vi "Master_Reader_StateMachine.vi"() -> ()   [LabVIEW 2016]
panel:
  in  "Data Directory Path":path
  in  "Directory Tree":string[](tree)
  out "arrof filesboi":path[](array[path])
  in  "Parse File / Folder":bool
  in  "target file / folder":path=path "C:/"
  in  "EXIT BUTTON":bool
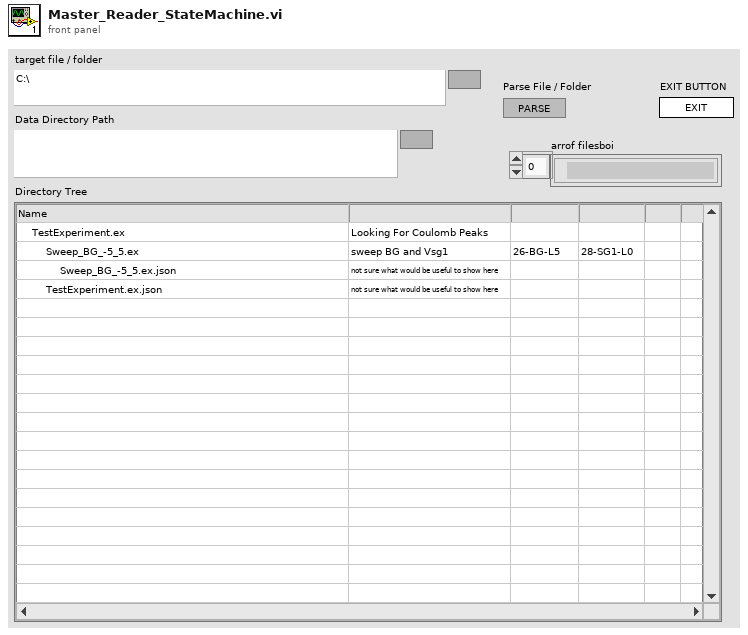
[diagram p1: front panel]
types:
  T1 = enum32{"invalid app kind", "Development System", "Run Time System", "Student Edition", "Embedded LabVIEW", "Evaluation", "Custom"}
  T2 = enum32{"Invalid", "Standard", "Closed", "Hidden", "Minimized", "Maximized"}
  T3 = cluster{"Core":cluster{"Current VI Reference":refnum<vi>, "Close Panel on Exit?":bool}, "array of files":path[], "Array of ITX Clusters ":cluster{"wave names":string[], "last modified timestamp":timestamp, "Comments":string, "Array of clusters of wave data":cluster{"wave data":dbl[]}[]}[], "target file / folder":path}
  T4 = cluster{"wave names":string[], "last modified timestamp":timestamp, "Comments":string, "Array of clusters of wave data":cluster{"wave data":dbl[]}[]}[]
  T5 = cluster{"Current VI Reference":refnum<vi>, "Close Panel on Exit?":bool}
  T6 = cluster{"wave names":string[], "last modified timestamp":timestamp, "Comments":string, "Array of clusters of wave data":cluster{"wave data":dbl[]}[]}
  T7 = typedef "imagedata.ctl" = cluster{"image type":i32, "image depth":i32, "image":u8[], "mask":u8[], "colors":u32[], "Rectangle":cluster{"left":i16, "top":i16, "right":i16, "bottom":i16}}
  T8 = cluster{"Left Cell String":string, "Child Text":string[], "Child Tag":string, "Item Indent":i32, "Child Only?":bool, "Glyph Index":i32}[]
  T9 = cluster{"Left Cell String":string, "Child Text":string[], "Child Tag":string, "Item Indent":i32, "Child Only?":bool, "Glyph Index":i32}
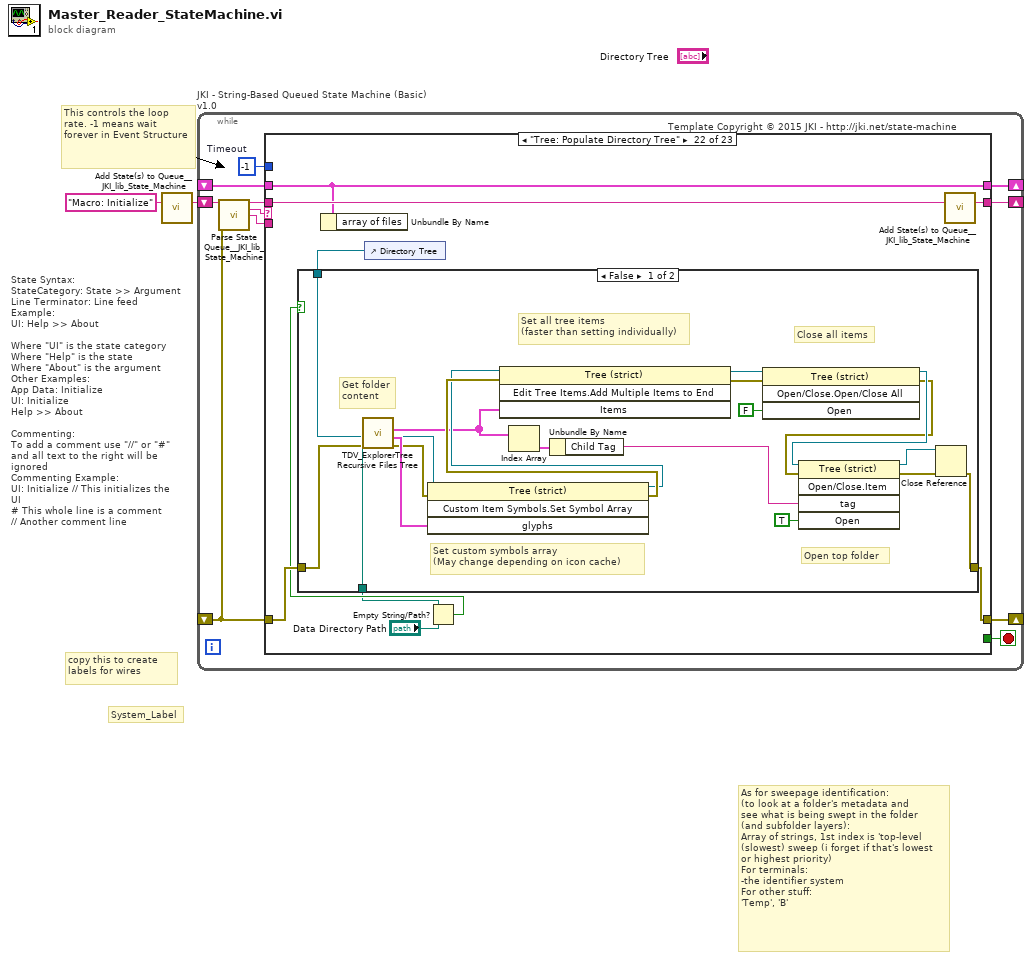
[diagram p0: block diagram]
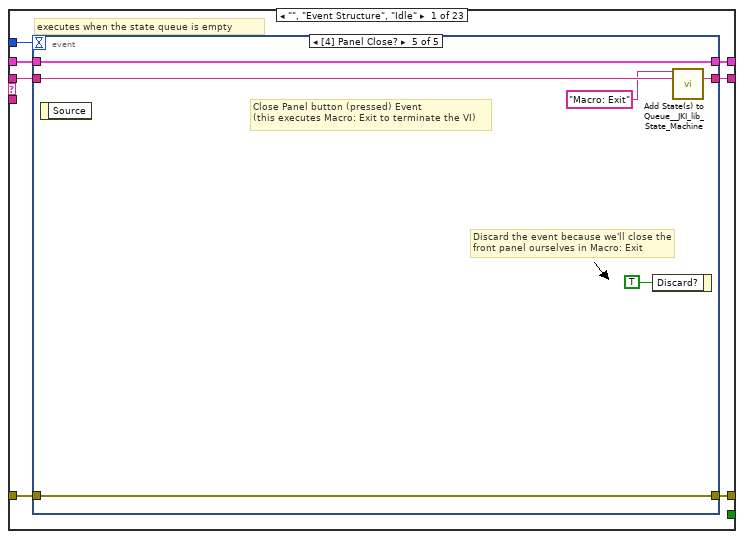
[diagram p2: hidden frame]
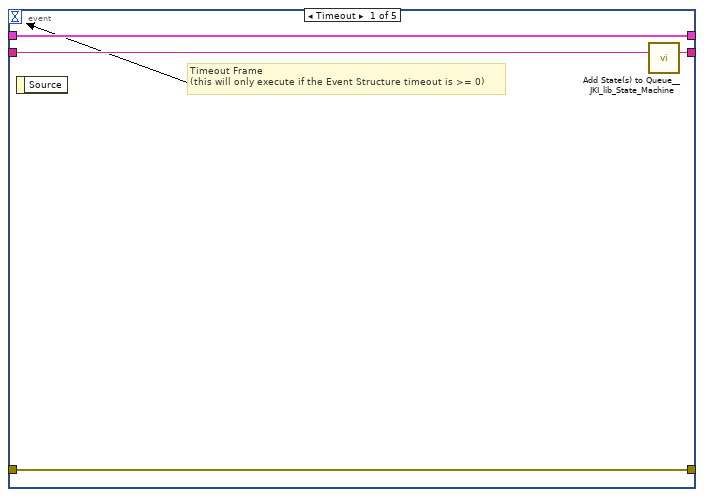
[diagram p3: hidden frame]
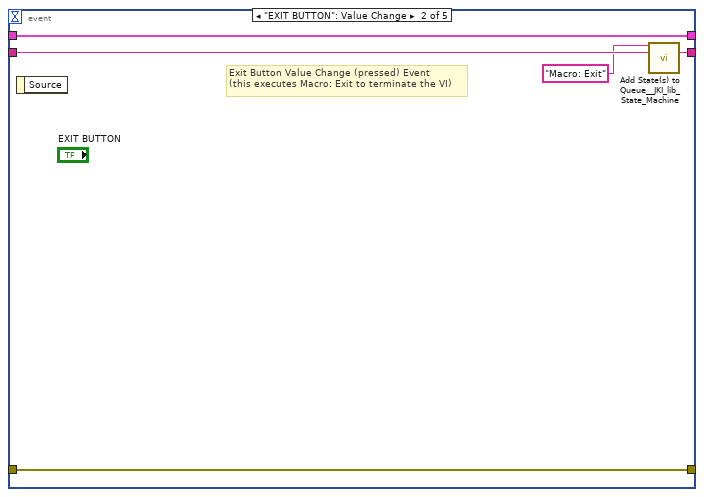
[diagram p4: hidden frame]
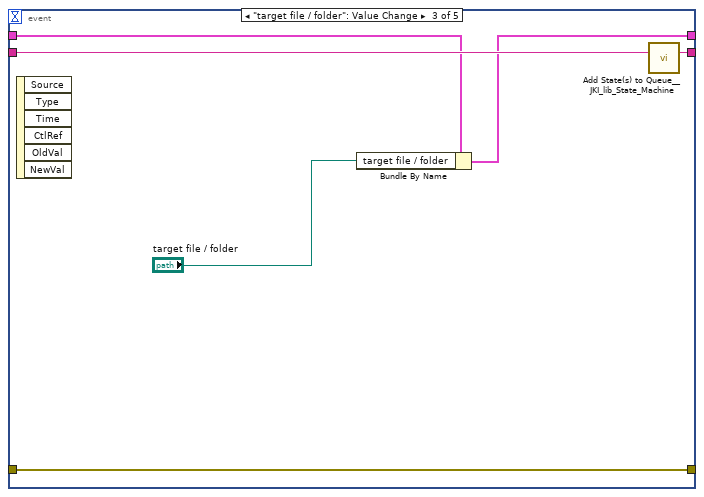
[diagram p5: hidden frame]
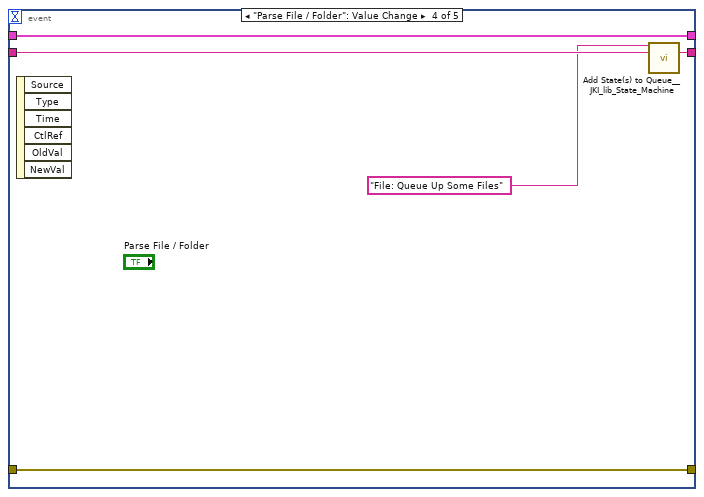
[diagram p6: hidden frame]
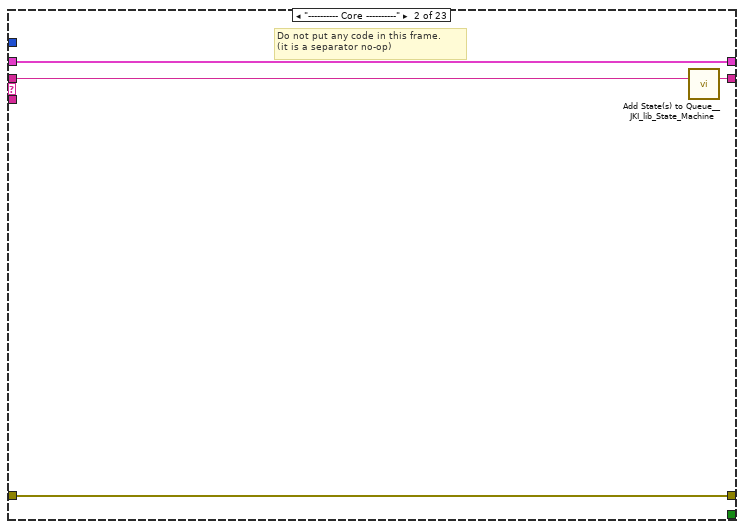
[diagram p7: hidden frame]
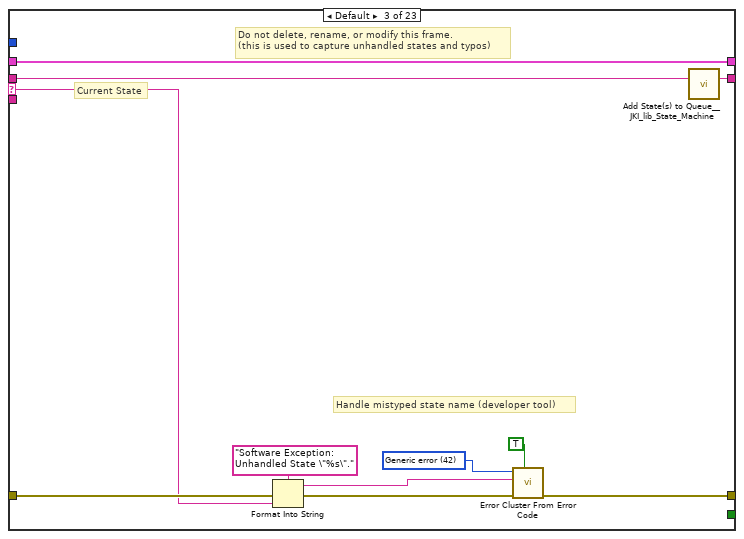
[diagram p8: hidden frame]
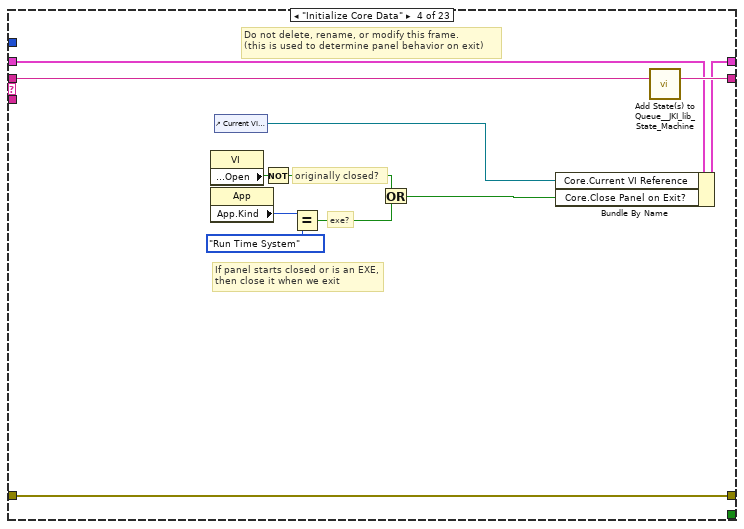
[diagram p9: hidden frame]
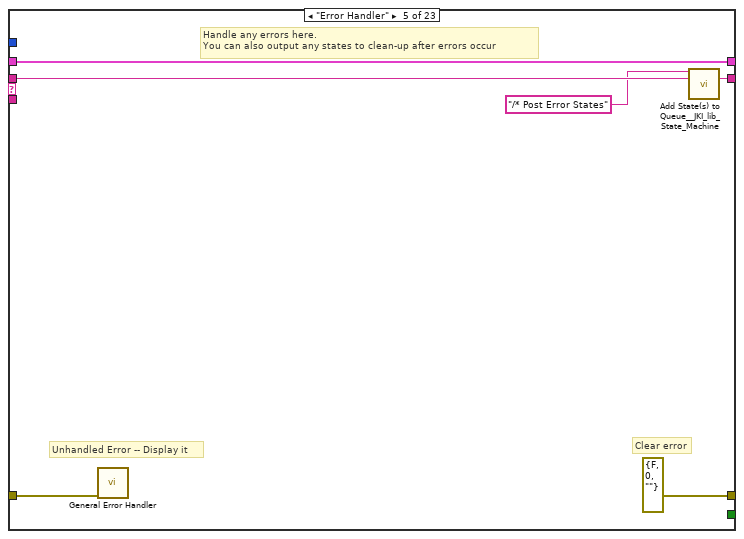
[diagram p10: hidden frame]
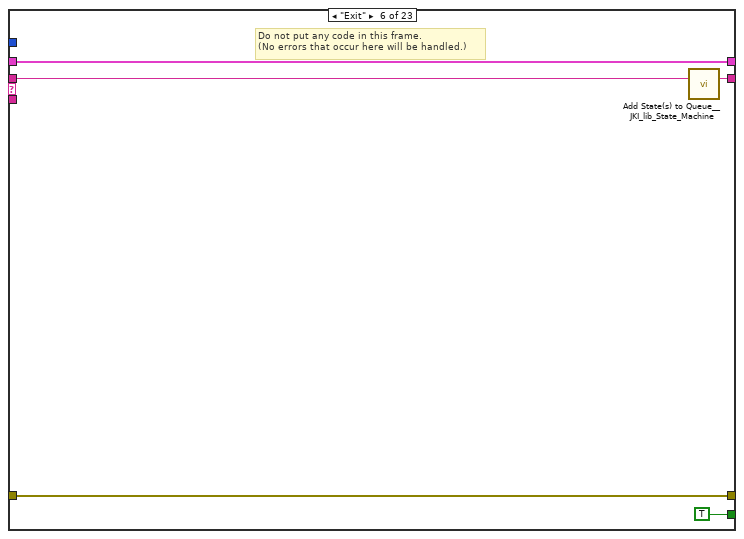
[diagram p11: hidden frame]
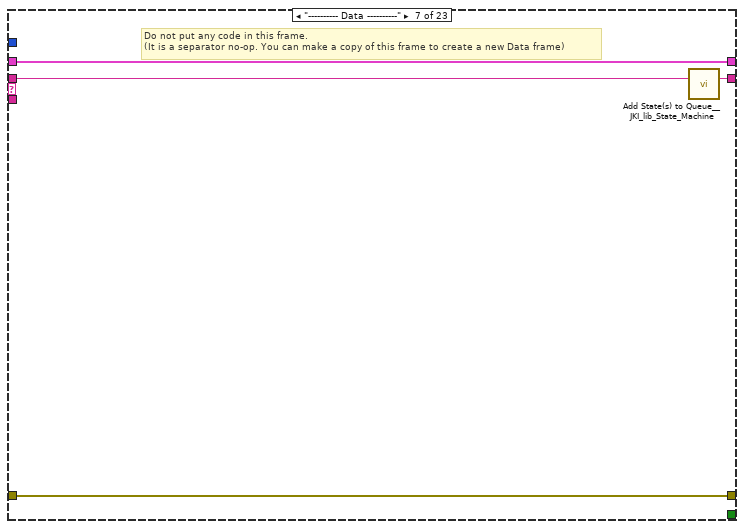
[diagram p12: hidden frame]
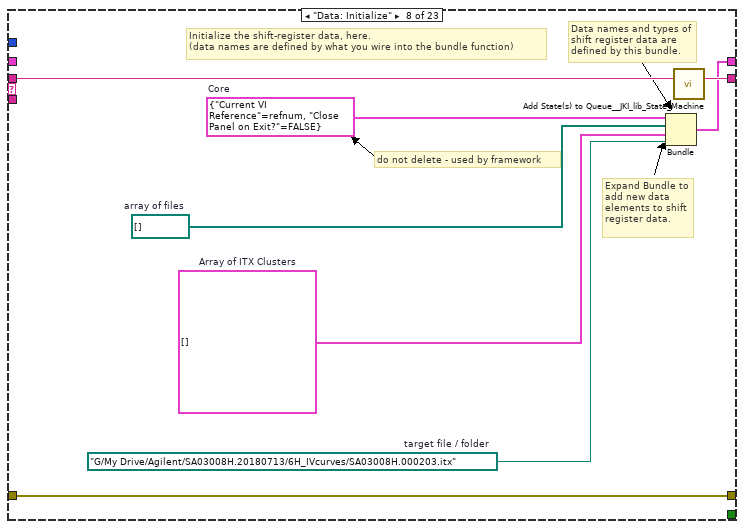
[diagram p13: hidden frame]
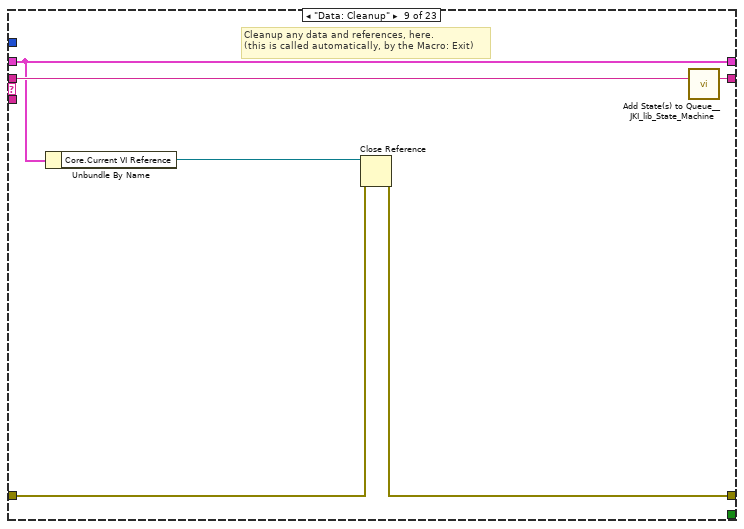
[diagram p14: hidden frame]
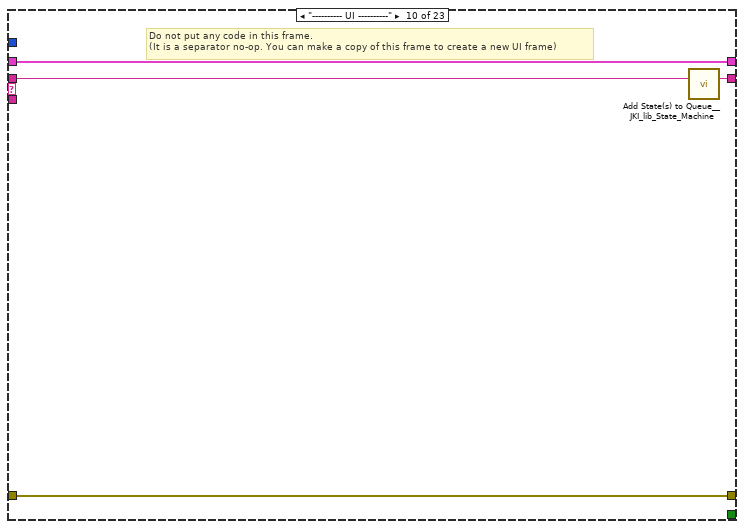
[diagram p15: hidden frame]
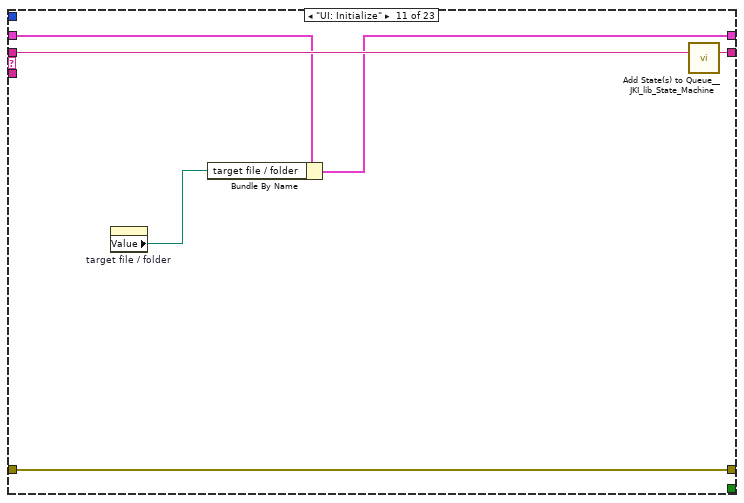
[diagram p16: hidden frame]
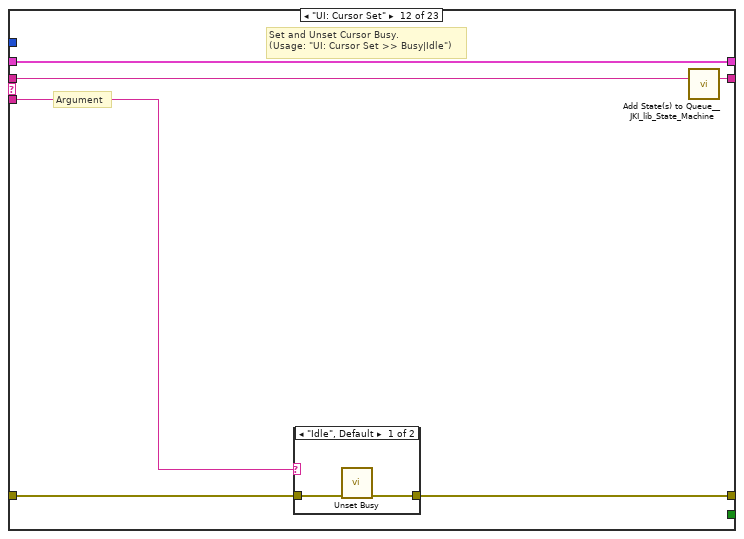
[diagram p17: hidden frame]
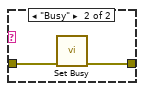
[diagram p18: hidden frame]
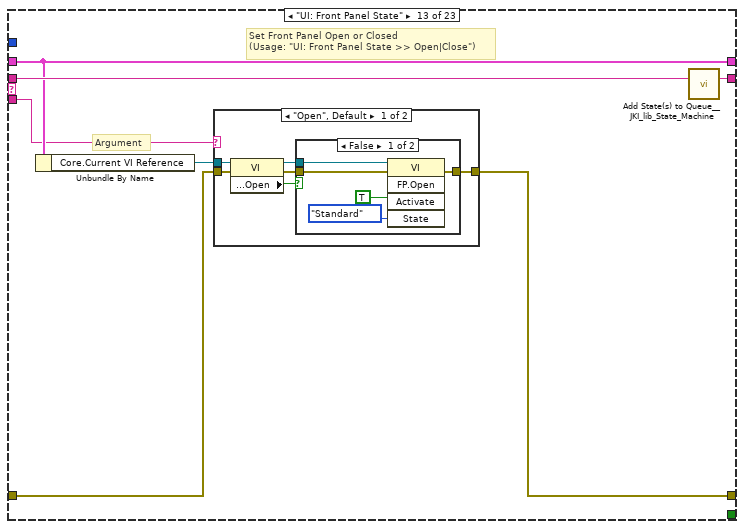
[diagram p19: hidden frame]
diagram:
  # "As for sweepage identification:\n(to look at a folder's metadata and\nsee what is being swept in the folder\n(and subfolder layers):\nArray of strings, 1st index is 'top-level\n(slowest) sweep (i forget if that's lowest\nor highest priority)\nFor terminals:\n-the identifier system\nFor other stuff:\n'Temp', 'B'"
  # "State Syntax:\nStateCategory: State >> Argument\nLine Terminator: Line feed\nExample:\nUI: Help >> About\n\nWhere \"UI\" is the state category\nWhere \"Help\" is the state\nWhere \"About\" is the argument\nOther Examples:\nApp Data: Initialize\nUI: Initialize\nHelp >> About\n\nCommenting:\nTo add a comment use \"//\" or \"#\" and all text to the right will be ignored\nCommenting Example:\nUI: Initialize // This initializes the UI\n# This whole line is a comment\n// Another comment line"
  # "copy this to create labels for wires"
  # "This controls the loop rate. -1 means wait forever in Event Structure"
  # "System_Label"
  n1 = call <vilib>:"Add State(s) to Queue__JKI_lib_State_Machine.vi"("State(s) in (\"\")"="Macro: Initialize") -> ("States Out"=w2:string)  [unwired: 14 in]
  n2 = while "JKI - String-Based Queued State Machine (Basic) v1.0" {
    shift-right: [w6] -> _
    shift-left: _ -> [w5]
    shift-right: [w9] -> _
    shift-left: _ -> [w3]
    shift-right: [w8] -> _
    shift-left: w2 -> [w10]
    stop <- w7 stop-if-true
    w4 = -1  # Timeout
    # "Template Copyright © 2015 JKI - http://jki.net/state-machine"
    n3 = call <vilib>:"Parse State Queue__JKI_lib_State_Machine.vi"("State Queue"=w10, "Error In (no error)"=w3) -> ("Remaining States"=w12:string, "Current State"=w13:string, "Arguments"=w11:string)  [unwired: 11 in]
    n4 = case shown="\"Tree: Populate Directory Tree\"" w13 {
      selector: w13 -> [_ _ w51 _ _ _ _ _ _ _ _ _ _ _ _ _ _ _ _ _ _ _ _]
      tunnel: w12 -> [w20 w50 w55 w73 w79 w84 w88 w96 w102 w106 w112 w118 w129 w155 w160 w170 w174 w184 w188 w196 w204 w212 w242]
      tunnel: w11 -> [_ _ _ _ _ _ _ _ _ _ _ w113 w123 _ _ _ _ _ _ _ _ _ _]
      tunnel: w5 -> [w18 w47 w53 w64 w76 w82 w85 _ w97 w103 w109 w116 w125 w152 w157 w167 w171 w179 w185 w191 w201 w206 w237]
      tunnel: [w17 w48 w57 w70 errorcluster {"status"=FALSE, "code"=0, "source"=""} ("error out") w81 w86 w93 w98 w104 w110 w114 w126 w153 w158 w168 w172 w181 w186 w192 w202 w207 w238] -> w9
      tunnel: w3 -> [w16 w48 w56 w70 w75 w81 w86 w93 w99 w104 w110 w115 w127 w153 w158 w168 w172 w182 w186 w193 w202 w209 w239]
      tunnel: [w19 w49 w54 w72 w78 w83 w87 w95 w101 w105 w111 w117 w128 w154 w159 w169 w173 w183 w187 w195 w203 w211 w241] -> w8
      tunnel: [_ _ _ _ _ TRUE _ _ _ _ _ _ _ _ _ _ _ _ _ _ _ _ _] -> w7
      tunnel: [w15 w47 w53 w71 w76 w82 w85 w94 w97 w103 w108 w116 w125 w152 w157 w167 w171 w178 w185 w190 w201 w206 w237] -> w6
      tunnel: w4 -> [w14 _ _ _ _ _ _ _ _ _ _ _ _ _ _ _ _ _ _ _ _ _ _]
      frame "", "Event Structure", "Idle" {
        # "executes when the state queue is empty"
        n5 = event shown="[4] Panel Close?" {
          selector: _ -> [_ _ _ _ _]
          dyn-events: _ -> [_ _ _ _ _]
          timeout: w14 -> [_ _ _ _ _]
          tunnel: w20 -> [w24 w29 w35 w40 w46]
          tunnel: [w23 w28 w34 w39 w45] -> w19
          tunnel: w18 -> [w21 w26 w32 w37 w43]
          tunnel: [w22 w27 w33 w38 w44] -> w17
          tunnel: w16 -> [w22 w27 w33 w38 w44]
          tunnel: [w21 w26 w31 w37 w43] -> w15
          event Timeout {
            # "Timeout Frame\n(this will only execute if the Event Structure timeout is >= 0)"
            n6 = event-data() -> ()  [unwired: 1 in, 1 out]
            n7 = call <vilib>:"Add State(s) to Queue__JKI_lib_State_Machine.vi"("State(s) in (\"\")"=w24) -> ("States Out"=w23:string)  [unwired: 14 in]
          }
          event "EXIT BUTTON": Value Change {
            # "Exit Button Value Change (pressed) Event\n(this executes Macro: Exit to terminate the VI)"
            n8 = event-data() -> ()  [unwired: 1 in, 1 out]
            n9 = call <vilib>:"Add State(s) to Queue__JKI_lib_State_Machine.vi"("State(s) in Front (\"\")"="Macro: Exit", "State(s) in (\"\")"=w29) -> ("States Out"=w28:string)  [unwired: 13 in]
          }
          event "target file / folder": Value Change {
            n10 = event-data() -> ()  [unwired: 1 in, 6 out]
            n11 = Bundle By Name(cluster=w32, "target file / folder"="target file / folder") -> (w31:T3)
            n12 = call <vilib>:"Add State(s) to Queue__JKI_lib_State_Machine.vi"("State(s) in (\"\")"=w35) -> ("States Out"=w34:string)  [unwired: 14 in]
          }
          event "Parse File / Folder": Value Change {
            n13 = event-data() -> ()  [unwired: 1 in, 6 out]
            n14 = call <vilib>:"Add State(s) to Queue__JKI_lib_State_Machine.vi"("State(s) in Front (\"\")"="File: Queue Up Some Files" ("State(s) in Front (\"\")"), "State(s) in (\"\")"=w40) -> ("States Out"=w39:string)  [unwired: 13 in]
          }
          event Panel Close? {
            # "Discard the event because we'll close the front panel ourselves in Macro: Exit"
            # "Close Panel button (pressed) Event\n(this executes Macro: Exit to terminate the VI)"
            n15 = event-data() -> ()  [unwired: 1 in, 1 out]
            n16 = event-data("Discard?"=TRUE) -> ()  [unwired: 1 in, 1 out]
            n17 = call <vilib>:"Add State(s) to Queue__JKI_lib_State_Machine.vi"("State(s) in Front (\"\")"="Macro: Exit", "State(s) in (\"\")"=w46) -> ("States Out"=w45:string)  [unwired: 13 in]
          }
        }
      }
      frame "---------- Core ----------" {
        # "Do not put any code in this frame.\n(it is a separator no-op)"
        n18 = call <vilib>:"Add State(s) to Queue__JKI_lib_State_Machine.vi"("State(s) in (\"\")"=w50) -> ("States Out"=w49:string)  [unwired: 14 in]
      }
      frame Default {
        w60 = 42 items=["No error", "Argument error", "Memory is full", "Out of zone", "End of file", "File already open", "Generic file I/O error", "File not found", "File permission error", "Disk is full", "Duplicate path", "Too many files open", "System feature not enabled", "Resource file not found", "Cannot add resource", "Resource not found", "Image not found", "Image memory error", "Pen does not exist", "Config type invalid", "Config token not found", "Config parse error", "Config memory error", "Bad external code format", "Bad external code offset", "External code not present", "Null window", "Destroy window error", "Null menu", "Print aborted", "Bad print record", "Print driver error", "Windows error during printing", "Memory error during printing", "Print dialog error", "Generic print error", "Invalid device refnum", "Device not found", "Device parameter error", "Device unit error", "Cannot open device", "Device call aborted", "Generic error", "Cancelled by user", "Object ID too low", "Object ID too high", "Object not in heap", "Unknown heap", "Unknown object (invalid DefProc)", "Unknown object (DefProc not in table)", "Message out of range", "Invalid (null) method", "Unknown message", "Manager call not supported", "Bad address", "Network operation in progress", "Network operation timed out", "Connection is busy", "Network attribute not supported", "Network error", "Address in use", "System out of memory", "Connection aborted", "Connection refused", "Not connected", "Already connected", "Connection closed", "Initialization error (interapplication manager)", "Bad occurrence", "Wait on unbound occurrence handler", "Occurrence queue overflow", "Datalog type conflict", "Unused", "Unrecognized type (interapplication manager)", "Memory corrupt", "Failed to make temporary DLL", "Old CIN version", "Drag socket not found", "Failed to load drop-object", "Failed to register OLE object", "Failed to release OLE object", "Format specifier type mismatch", "Unknown format specifier", "Too few format specifiers", "Too many format specifiers", "Scan failed", "Newer CIN version", "Error converting to variant", "Runtime menu error", "Password tampered", "Variant attribute not found", "Incompatible variant data type", "Event data is not available", "Event Store is not present", "Occurrence is not found", "Event Queue is not created", "Event info is not available", "Refnum passed is NULL", "Error retrieving Class GUID", "Error retrieving CoClass GUID", "Error retrieving TypeLib GUID.", "Bad built application magic bytes.", "Specific driver is different from the specific driver associated with the Logical Name.", "There is no session opened to the class driver.", "Max Error", "MAX - Error with config objects", "MAX - Error loading configuration", "MAX - Group not supported"]
        # "Current State"
        # "Do not delete, rename, or modify this frame.\n(this is used to capture unhandled states and typos)"
        # "Handle mistyped state name (developer tool)"
        n19 = Format Into String(format string="Software Exception: Unhandled State \"%s\"." ("message"), error in=w56, w51) -> (resulting string=w59:string, error out=w58:errorcluster)  [unwired: 1 in]
        n20 = call <vilib>:"Error Cluster From Error Code.vi"("show call chain? (False)"=TRUE, "error in (no error)"=w58, "error message (\"\")"=w59, "error code (0)"=w60) -> ("error out"=w57:errorcluster)  [unwired: 5 in]
        n21 = call <vilib>:"Add State(s) to Queue__JKI_lib_State_Machine.vi"("State(s) in (\"\")"=w55) -> ("States Out"=w54:string)  [unwired: 14 in]
      }
      frame "Initialize Core Data" {
        # "Do not delete, rename, or modify this frame.\n(this is used to determine panel behavior on exit)"
        # "originally closed?"
        # "exe?"
        # "If panel starts closed or is an EXE, then close it when we exit"
        n22 = property class="VI"() -> ("Front Panel.Open"=w69:bool)  [unwired: 2 in, 2 out]
        n23 = property class="App"() -> ("App.Kind"=w68:T1)  [unwired: 2 in, 2 out]
        n24 = control-ref of="Current VI Reference"() -> (w62:refnum<vi>)
        n25 = Not(x=w69) -> (.not. x?=w66:bool)
        n26 = Equal?(x=w68, y=T1."Run Time System" ("Application:Kind")) -> (x = y?=w65:bool)
        n27 = Or(x=w66, y=w65) -> (x .or. y?=w63:bool)
        n28 = Bundle By Name(cluster=w64, "Core.Current VI Reference"=w62, "Core.Close Panel on Exit?"=w63) -> (w71:T3)
        n29 = call <vilib>:"Add State(s) to Queue__JKI_lib_State_Machine.vi"("State(s) in (\"\")"=w73) -> ("States Out"=w72:string)  [unwired: 14 in]
      }
      frame "Error Handler" {
        # "Unhandled Error -- Display it"
        # "Handle any errors here.\nYou can also output any states to clean-up after errors occur"
        # "Clear error"
        n30 = call <vilib>:"General Error Handler.vi"("error in (no error)"=w75) -> ()  [unwired: 10 in, 5 out]
        n31 = call <vilib>:"Add State(s) to Queue__JKI_lib_State_Machine.vi"("State(s) in Front (\"\")"="/* Post Error States", "State(s) in (\"\")"=w79) -> ("States Out"=w78:string)  [unwired: 13 in]
      }
      frame "Exit" {
        # "Do not put any code in this frame.\n(No errors that occur here will be handled.)"
        n32 = call <vilib>:"Add State(s) to Queue__JKI_lib_State_Machine.vi"("State(s) in (\"\")"=w84) -> ("States Out"=w83:string)  [unwired: 14 in]
      }
      frame "---------- Data ----------" {
        # "Do not put any code in this frame.\n(It is a separator no-op. You can make a copy of this frame to create a new Data frame)"
        n33 = call <vilib>:"Add State(s) to Queue__JKI_lib_State_Machine.vi"("State(s) in (\"\")"=w88) -> ("States Out"=w87:string)  [unwired: 14 in]
      }
      frame "Data: Initialize" {
        w89 = path "G:/My Drive/Agilent/SA03008H.20180713/6H_IVcurves/SA03008H.000203.itx"  # target file / folder
        w90 = T4 []  # Array of ITX Clusters
        w91 = path[] []  # array of files
        w92 = T5 {"Current VI Reference"=refnum, "Close Panel on Exit?"=FALSE}  # Core
        # "do not delete - used by framework"
        # "Expand Bundle to add new data elements to shift register data."
        # "Data names and types of shift register data are defined by this bundle."
        # "Initialize the shift-register data, here.\n(data names are defined by what you wire into the bundle function)"
        n34 = Bundle("Core"=w92, "array of files"=w91, "Array of ITX Clusters"=w90, "target file / folder"=w89) -> (w94:T3)  [unwired: 1 in]
        n35 = call <vilib>:"Add State(s) to Queue__JKI_lib_State_Machine.vi"("State(s) in (\"\")"=w96) -> ("States Out"=w95:string)  [unwired: 14 in]
      }
      frame "Data: Cleanup" {
        # "Cleanup any data and references, here.\n(this is called automatically, by the Macro: Exit)"
        n36 = Unbundle By Name(w97) -> ("Core.Current VI Reference"=w100:refnum<vi>)
        n37 = Close Reference(reference=w100, error in (no error)=w99) -> (error out=w98:errorcluster)
        n38 = call <vilib>:"Add State(s) to Queue__JKI_lib_State_Machine.vi"("State(s) in (\"\")"=w102) -> ("States Out"=w101:string)  [unwired: 14 in]
      }
      frame "---------- UI ----------" {
        # "Do not put any code in this frame.\n(It is a separator no-op. You can make a copy of this frame to create a new UI frame)"
        n39 = call <vilib>:"Add State(s) to Queue__JKI_lib_State_Machine.vi"("State(s) in (\"\")"=w106) -> ("States Out"=w105:string)  [unwired: 14 in]
      }
      frame "UI: Initialize" {
        n40 = property on="target file / folder" class="Path"() -> ("Value"=w107:path)  [unwired: 2 in, 2 out]
        n41 = Bundle By Name(cluster=w109, "target file / folder"=w107) -> (w108:T3)
        n42 = call <vilib>:"Add State(s) to Queue__JKI_lib_State_Machine.vi"("State(s) in (\"\")"=w112) -> ("States Out"=w111:string)  [unwired: 14 in]
      }
      frame "UI: Cursor Set" {
        # "Argument"
        # "Set and Unset Cursor Busy.\n(Usage: \"UI: Cursor Set >> Busy|Idle\")"
        n43 = case shown="\"Idle\", Default" w113 {
          tunnel: w115 -> [w120 w122]
          tunnel: [w119 w121] -> w114
          frame "Idle", Default {
            n44 = call <vilib>:"Unset Busy.vi"("error in (no error)"=w120) -> ("error out"=w119:errorcluster)  [unwired: 10 in]
          }
          frame "Busy" {
            n45 = call <vilib>:"Set Busy.vi"("error in (no error)"=w122) -> ("error out"=w121:errorcluster)  [unwired: 9 in, 1 out]
          }
        }
        n46 = call <vilib>:"Add State(s) to Queue__JKI_lib_State_Machine.vi"("State(s) in (\"\")"=w118) -> ("States Out"=w117:string)  [unwired: 14 in]
      }
      frame "UI: Front Panel State" {
        # "Argument"
        # "Set Front Panel Open or Closed\n(Usage: \"UI: Front Panel State >> Open|Close\")"
        n47 = Unbundle By Name(w125) -> ("Core.Current VI Reference"=w124:refnum<vi>)
        n48 = case shown="\"Open\", Default" w123 {
          tunnel: w127 -> [w133 w146]
          tunnel: [w135 w147] -> w126
          tunnel: w124 -> [w134 w144]
          frame "Open", Default {
            n49 = property class="VI"(reference=w134, error in=w133) -> (reference out=w131:refnum<vi>, error out=w132:errorcluster, "Front Panel.Open"=w130:bool)
            n50 = case shown="False" w130 {
              tunnel: [w138 w141] -> w135
              tunnel: w132 -> [w137 w141]
              tunnel: w131 -> [w136 _]
              frame False {
                n51 = invoke class="VI" method="FP.Open"(reference=w136, error in=w137, "Activate"=TRUE, "State"=T2."Standard") -> (error out=w138:errorcluster)  [unwired: 1 in, 4 out]
              }
              frame True {
              }
            }
          }
          frame "Close" {
            n52 = property class="VI"(reference=w144, error in=w146) -> (reference out=w143:refnum<vi>, error out=w145:errorcluster, "Front Panel.Open"=w142:bool)
            n53 = case shown="True" w142 {
              tunnel: [w148 w151] -> w147
              tunnel: w145 -> [w148 w150]
              tunnel: w143 -> [_ w149]
              frame False {
              }
              frame True {
                n54 = invoke class="VI" method="FP.Close"(reference=w149, error in=w150) -> (error out=w151:errorcluster)  [unwired: 1 in, 2 out]
              }
            }
          }
        }
        n55 = call <vilib>:"Add State(s) to Queue__JKI_lib_State_Machine.vi"("State(s) in (\"\")"=w129) -> ("States Out"=w128:string)  [unwired: 14 in]
      }
      frame "---------- Macro ----------" {
        # "Do not put any code in this frame.\n(It is a separator no-op. You can make a copy of this frame to create a new Macro frame)"
        n56 = call <vilib>:"Add State(s) to Queue__JKI_lib_State_Machine.vi"("State(s) in (\"\")"=w155) -> ("States Out"=w154:string)  [unwired: 14 in]
      }
      frame "Macro: Initialize" {
        w156 = "Data: Initialize\nInitialize Core Data\nTree: Clear Directory Tree\nTree: Populate Directory Tree\nUI: Initialize\nUI: Front Panel State >> Open"  # Data: Initialize Initialize Core Data Tree: Clear Directory Tree Tree: Populate Directory Tree UI: Initialize UI: Front Panel State >> Open
        # "Initialization Macro\n(This is called once, when the VI starts)"
        n57 = call <vilib>:"Add State(s) to Queue__JKI_lib_State_Machine.vi"("State(s) in Front (\"\")"=w156, "State(s) in (\"\")"=w160) -> ("States Out"=w159:string)  [unwired: 13 in]
      }
      frame "Macro: Exit" {
        # "Exit Macro\n(This is called once, when the VI exits)"
        n58 = Unbundle By Name(w167) -> ("Core.Close Panel on Exit?"=w166:bool)
        n59 = Select(t="UI: Front Panel State >> Close", s=w166, f="") -> (s? t:f=w163:string)
        n60 = call <vilib>:"Add State(s) to Queue__JKI_lib_State_Machine.vi"("State(s) in (\"\")"=w163, "State(s) at Back (\"\")"="Data: Cleanup\nExit") -> ("States Out"=w161:string)  [unwired: 13 in]
        n61 = call <vilib>:"Add State(s) to Queue__JKI_lib_State_Machine.vi"("State(s) in Front (\"\")"=w161, "State(s) in (\"\")"=w170) -> ("States Out"=w169:string)  [unwired: 13 in]
      }
      frame "---------- File ----------" {
        # "Template Separator\n(You can make a copy of, or modify, this frame)"
        n62 = call <vilib>:"Add State(s) to Queue__JKI_lib_State_Machine.vi"("State(s) in (\"\")"=w174) -> ("States Out"=w173:string)  [unwired: 14 in]
      }
      frame "File: Queue Up Some Files" {
        # "can accept a file or folder"
        n63 = Unbundle By Name(w179) -> ("target file / folder"=w180:path, "array of files"=w177:path[])
        n64 = call "Path_to_Array_Of_Filepaths.vi"("error in (no error)"=w182, "File or Folder Path"=w180) -> ("error out"=w181:errorcluster, "array of files"=w176:path[])  [unwired: 7 in, 1 out]
        n65 = Build Array (concatenate)(w177, w176) -> (w175:path[])
        "arrof filesboi" <- w175
        n66 = Bundle By Name(cluster=w179, "array of files"=w175) -> (w178:T3)
        n67 = call <vilib>:"Add State(s) to Queue__JKI_lib_State_Machine.vi"("State(s) in (\"\")"=w184) -> ("States Out"=w183:string)  [unwired: 14 in]
      }
      frame "---------- Wave ----------" {
        # "Template Separator\n(You can make a copy of, or modify, this frame)"
        n68 = call <vilib>:"Add State(s) to Queue__JKI_lib_State_Machine.vi"("State(s) in (\"\")"=w188) -> ("States Out"=w187:string)  [unwired: 14 in]
      }
      frame "Wave: Grab Wave Data From File Array" {
        n69 = Unbundle By Name(w191) -> ("array of files"=w194:path[])
        n70 = for {
          tunnel: w194 -> [w200] mode=indexing
          shift-right: [w198] -> w192
          shift-left: w193 -> [w199]
          tunnel: [w197] -> w189 mode=indexing
          n71 = call "Single_ITX_to_Wave_Info.vi"("error in (no error)"=w199, "Path"=w200) -> ("error out"=w198:errorcluster, "Single ITX cluster"=w197:T6)  [unwired: 8 in]
        }
        n72 = Bundle By Name(cluster=w191, "Array of ITX Clusters"=w189) -> (w190:T3)
        n73 = call <vilib>:"Add State(s) to Queue__JKI_lib_State_Machine.vi"("State(s) in (\"\")"=w196) -> ("States Out"=w195:string)  [unwired: 14 in]
      }
      frame "---------- Tree ----------" {
        # "Template Separator\n(You can make a copy of, or modify, this frame)"
        n74 = call <vilib>:"Add State(s) to Queue__JKI_lib_State_Machine.vi"("State(s) in (\"\")"=w204) -> ("States Out"=w203:string)  [unwired: 14 in]
      }
      frame "Tree: Populate Directory Tree" {
        n75 = Unbundle By Name(w206) -> ()  [unwired: 1 out]
        n76 = control-ref of="Directory Tree"() -> (w210:refnum<vi>)
        n77 = Empty String/Path?(string/path="Data Directory Path") -> (empty?=w208:bool)
        n78 = case shown="False" w208 {
          tunnel: w210 -> [w214 _]
          tunnel: "Data Directory Path" -> [w231 _]
          tunnel: w209 -> [w213 w233]
          tunnel: [w215 w232] -> w207
          frame False {
            # "Set custom symbols array\n(May change depending on icon cache)"
            # "Open top folder"
            # "Close all items"
            # "Set all tree items\n(faster than setting individually)"
            # "Get folder\ncontent"
            n79 = call "TDV_ExplorerTree Recursive Files Tree.vi"("error in (no error)"=w213, "Folder Path"=w231) -> ("error out"=w217:errorcluster, "Glyphs"=w230:T7[], "Items"=w223:T8)  [unwired: 6 in, 1 out]
            n80 = invoke class="Tree (strict)" method="Custom Item Symbols.Set Symbol Array"(reference=w214, error in=w217, "glyphs"=w230) -> (reference out=w228:refnum<vi>, error out=w229:errorcluster)  [unwired: 1 in, 2 out]
            n81 = invoke class="Tree (strict)" method="Edit Tree Items.Add Multiple Items to End"(reference=w228, error in=w229, "Items"=w223) -> (reference out=w226:refnum<vi>, error out=w227:errorcluster)  [unwired: 1 in, 2 out]
            n82 = Index Array(array=w223) -> (element=w222:T9)  [unwired: 1 in]
            n83 = Unbundle By Name(w222) -> ("Child Tag"=w221:string)
            n84 = invoke class="Tree (strict)" method="Open/Close.Open/Close All"(reference=w226, error in=w227, "Open"=FALSE ("Open?")) -> (reference out=w224:refnum<vi>, error out=w216:errorcluster)  [unwired: 1 in, 2 out]
            n85 = invoke class="Tree (strict)" method="Open/Close.Item"(reference=w224, error in=w216, "tag"=w221, "Open"=TRUE ("Open?")) -> (reference out=w218:refnum<vi>, error out=w219:errorcluster)  [unwired: 1 in, 3 out]
            n86 = Close Reference(reference=w218, error in (no error)=w219) -> (error out=w215:errorcluster)
          }
          frame True {
            n87 = call <vilib>:"Error Cluster From Error Code.vi"("error in (no error)"=w233, "error message (\"\")"="Folder Path cannot be empty" ("source"), "error code (0)"=5000) -> ("error out"=w232:errorcluster)  [unwired: 6 in]
          }
        }
        n88 = call <vilib>:"Add State(s) to Queue__JKI_lib_State_Machine.vi"("State(s) in (\"\")"=w212) -> ("States Out"=w211:string)  [unwired: 14 in]
      }
      frame "Tree: Clear Directory Tree" {
        # "Delete all tree items"
        n89 = Unbundle By Name(w237) -> ()  [unwired: 1 out]
        n90 = control-ref of="Directory Tree"() -> (w240:refnum<vi>)
        n91 = invoke class="Tree (strict)" method="Edit Tree Items.Delete"(reference=w240, error in=w239, "Delete Children"=TRUE ("Delete Children?")) -> (error out=w238:errorcluster)  [unwired: 2 in, 4 out]
        n92 = call <vilib>:"Add State(s) to Queue__JKI_lib_State_Machine.vi"("State(s) in (\"\")"=w242) -> ("States Out"=w241:string)  [unwired: 14 in]
      }
    }
  }
